vi "InstrumentationU6Mk2.vi"() -> ()   [LabVIEW 2021]
panel:
  out "Waveform Chart 5":dbl(graph)
  out "Waveform Chart 4":dbl(graph)
  out "Waveform Chart 3":dbl(graph)
  out "Waveform Chart 2":dbl(graph)
  out "Waveform Chart":dbl(graph)
  in  "Log Values":bool
  in  "file name":string
  in  "file path":path
  in  "Binary":bool
  in  "SettlingFactor":i32
  in  "Ranges":string[](array[string])=["LJ_rgBIP10V", "LJ_rgBIP10V", "LJ_rgBIPP01V", "LJ_rgBIPP01V"]
  out "Values Read":dbl[](array[numeric]) format="%.6f"
  out "Error Message":string
  in  "Resolution":i32
  out "error out":errorcluster
  # "Aquires multiple analog input channels over USB from the first found U6.\n\nThis uses eAddGoGet from the UD driver, rather than the LabVIEW utility AddS-Go-Get.vi.  The utility\nVI has better/easier error handling and is normally preferred, but eAddGoGet is a single call to the UD driver\nso often preferred if you will have parallel driver calls to the same handle within the same thread (none of\nour examples do this)."
  # "LJ_rgBIP10V\nLJ_rgBIP1V\nLJ_rgBIPP1V\nLJ_rgBIPP01V"
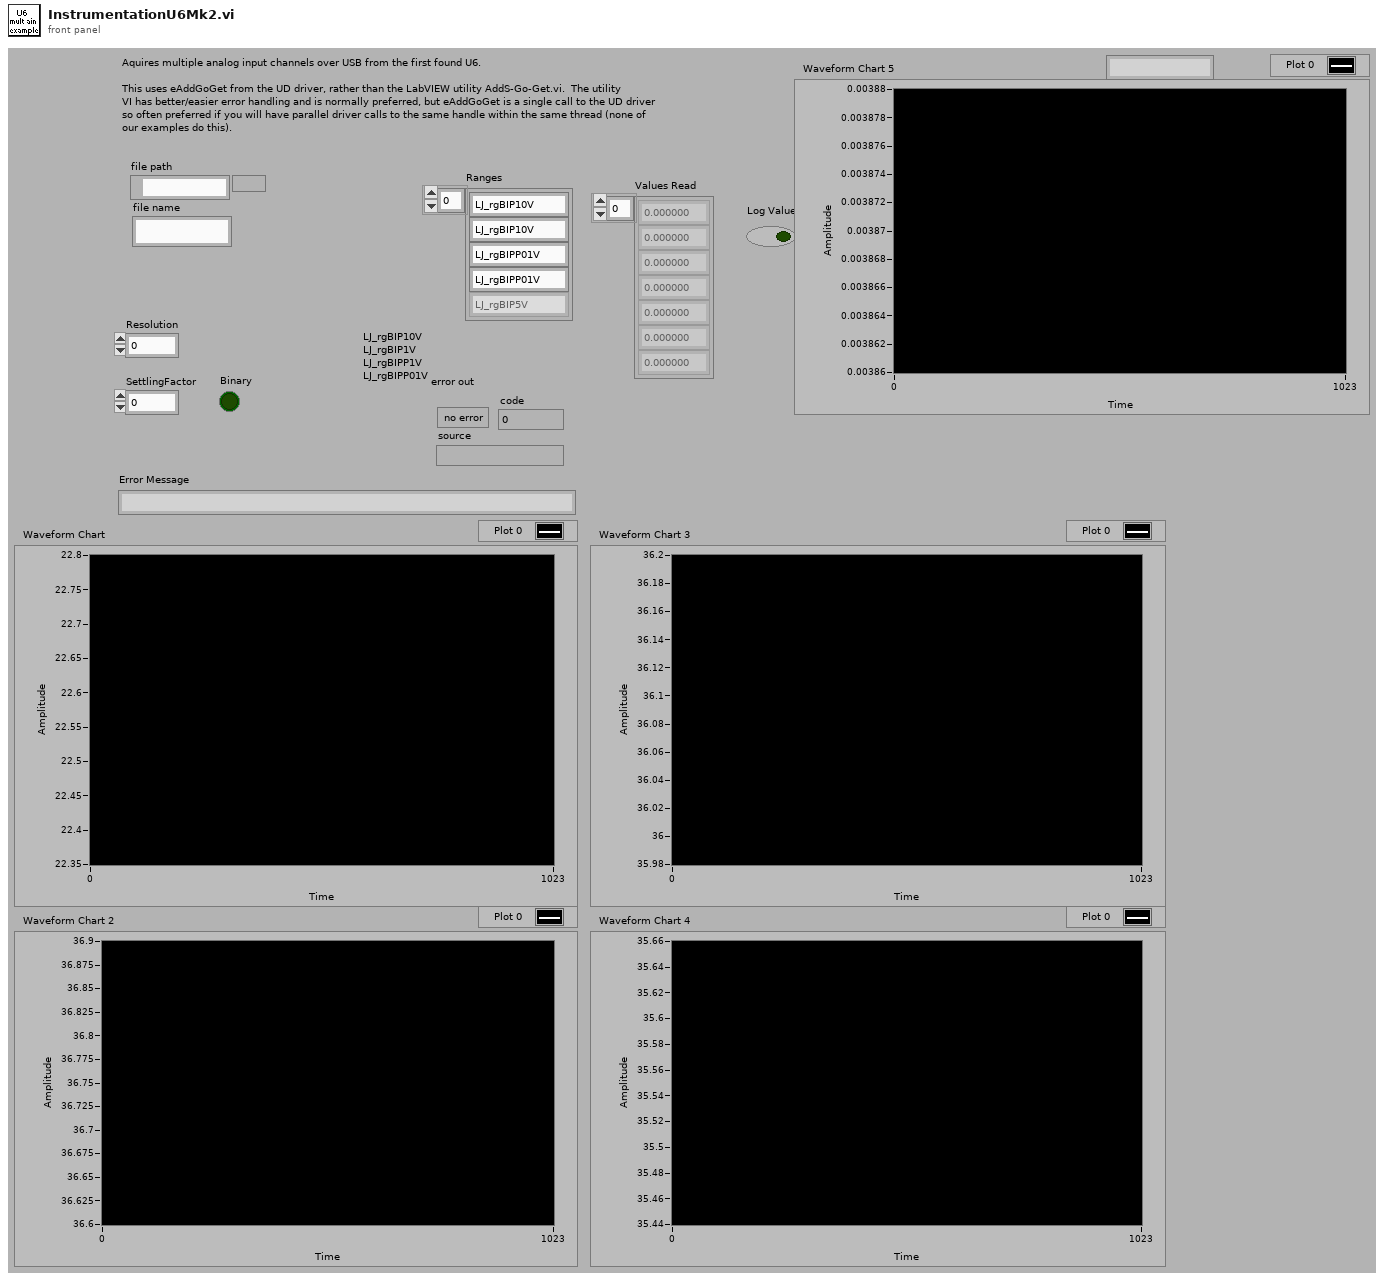
[diagram p1: front panel]
types:
  T1 = enum16{"open", "open or create", "create or replace", "create", "open (read-only)"}
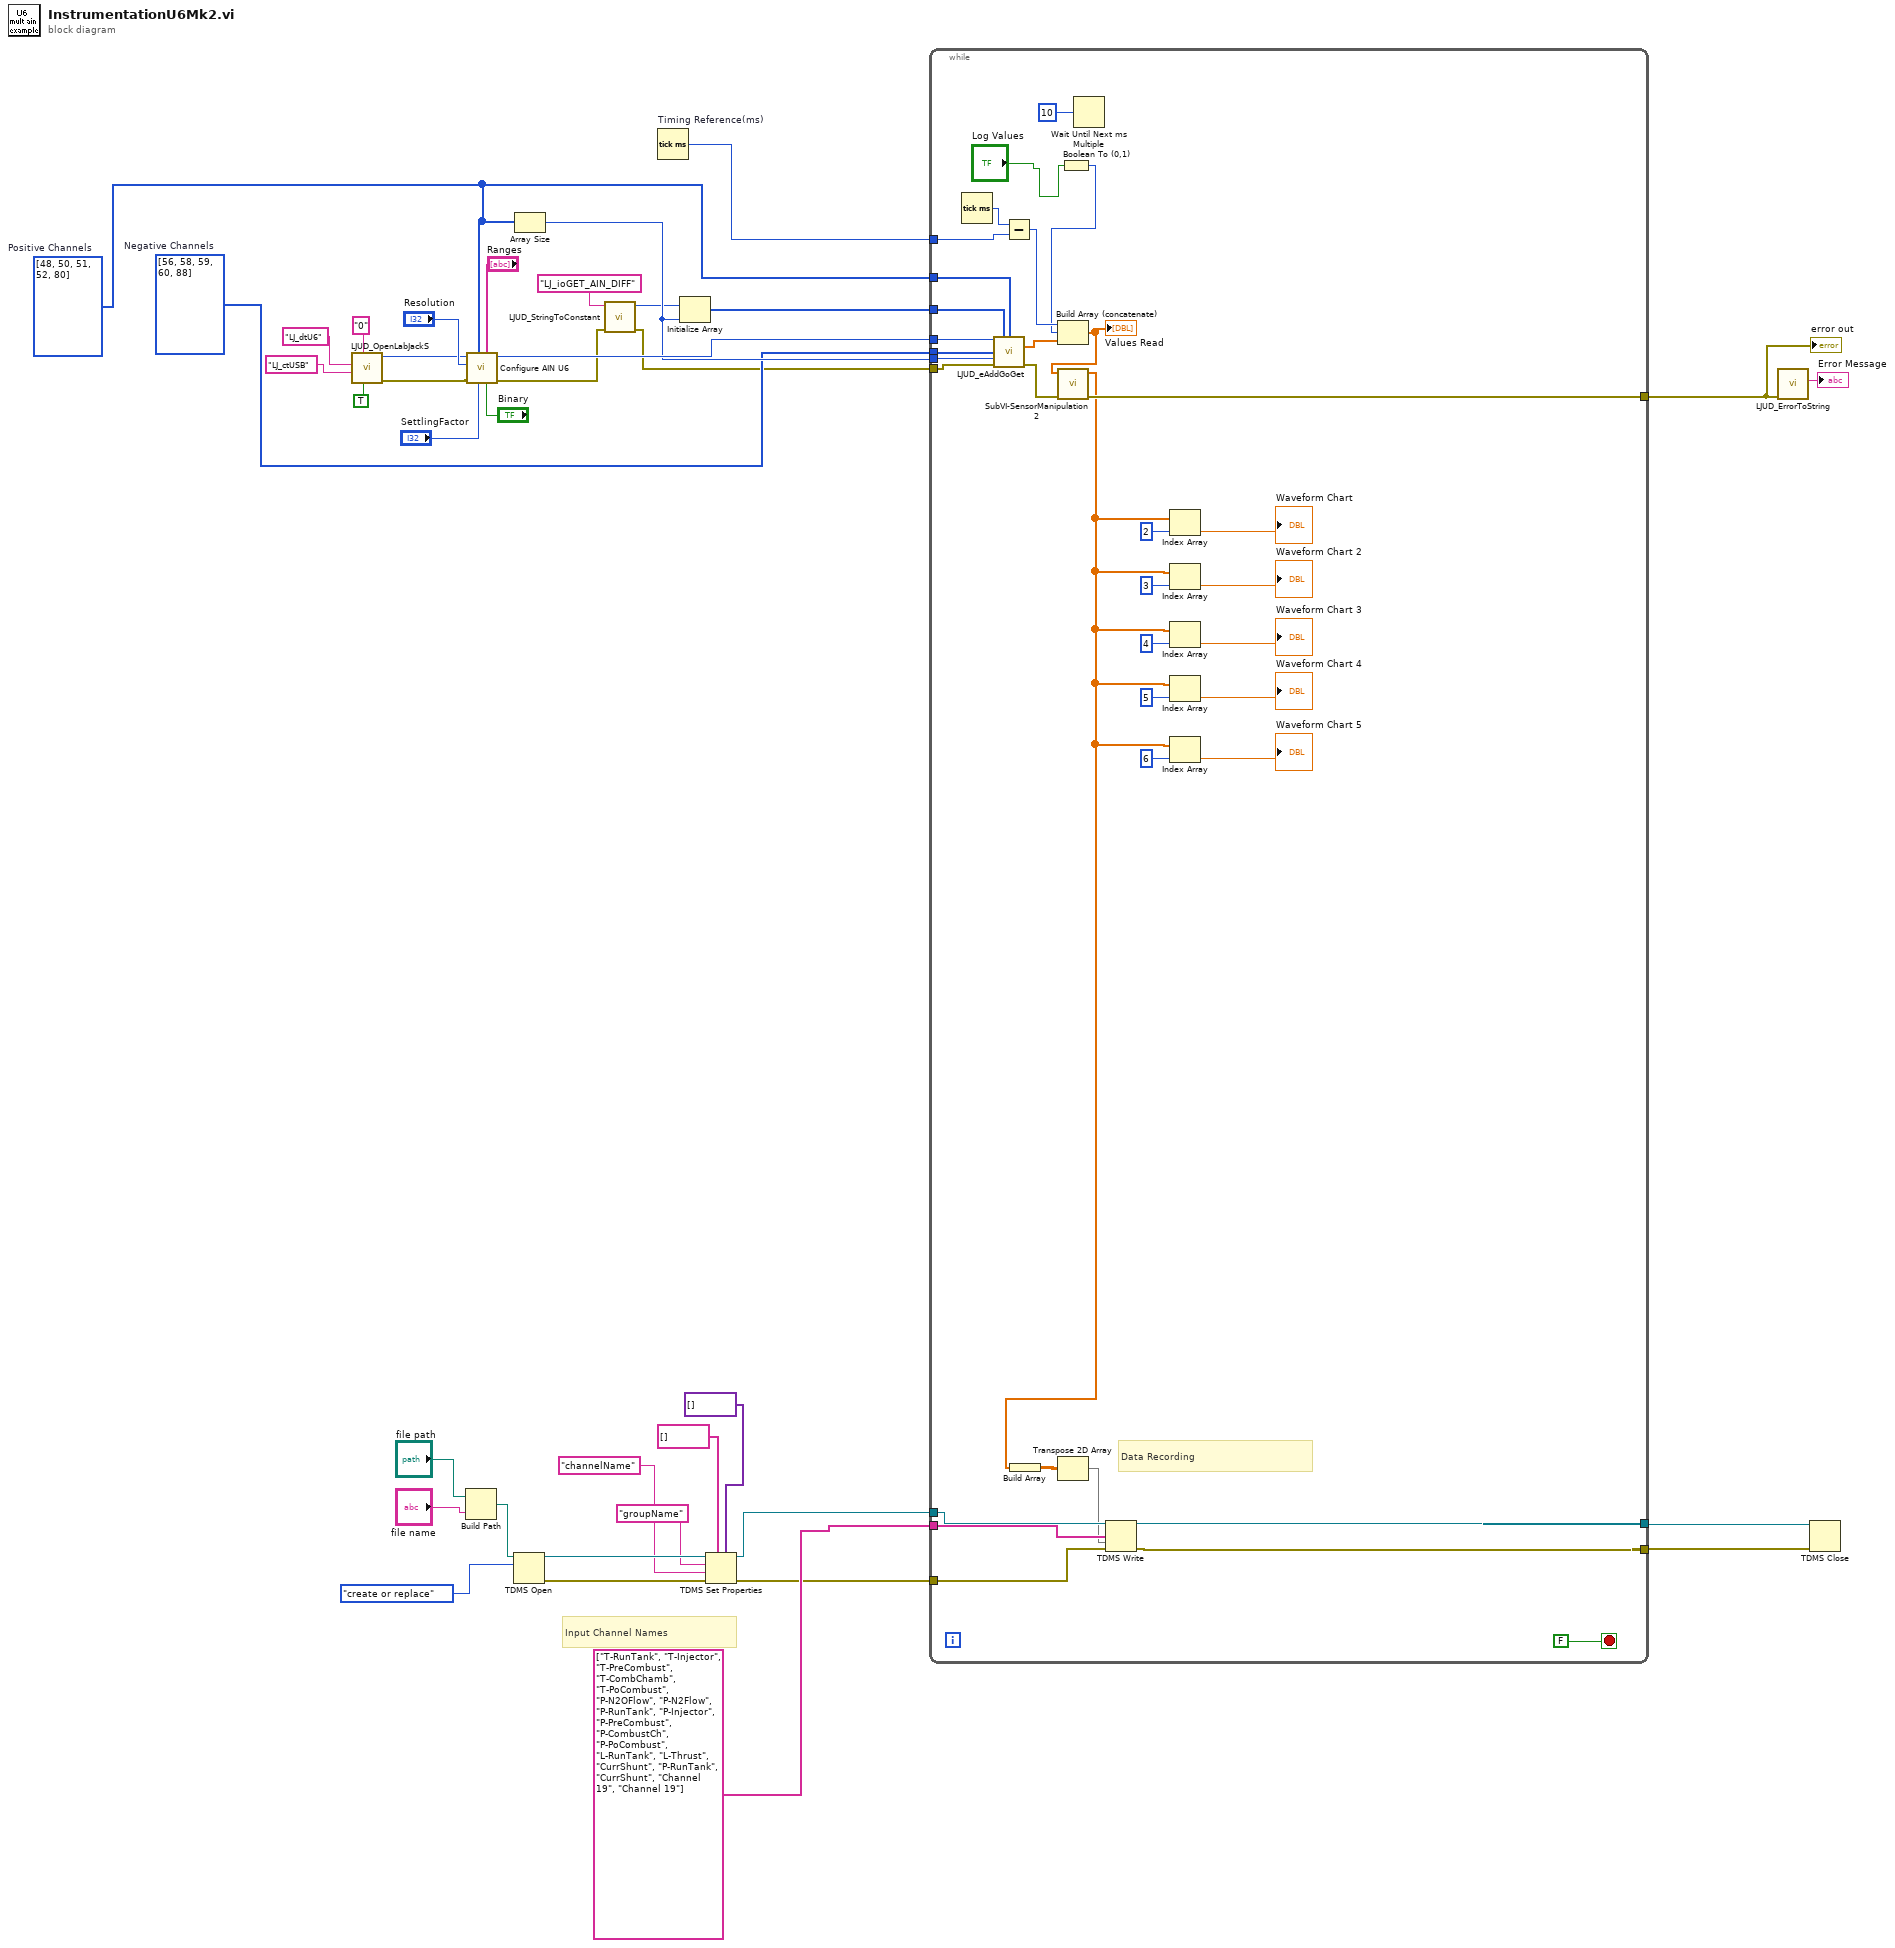
[diagram p0: block diagram]
diagram:
  w19 = i32[] [56, 58, 59, 60, 88]  # Negative Channels
  w18 = i32[] [48, 50, 51, 52, 80]  # Positive Channels
  # "Input Channel Names"
  n1 = call "LJUD_OpenLabJackS.vi"("FirstFound"=TRUE, "Address"="0", "ConnectionType"="LJ_ctUSB", "DeviceType"="LJ_dtU6") -> ("error out"=w28:errorcluster, "Handle"=w29:i32)  [unwired: 5 in, 1 out]
  n2 = Build Path(base path="file path", name or relative path="file name") -> (appended path=w12:path)
  n3 = call "Configure AIN U6.vi"("Binary"="Binary", "Ranges"="Ranges", "SettlingFactor"="SettlingFactor", "Positive Channels"=w18, "error in"=w28, "Resolution"="Resolution", "Handle In"=w29) -> ("error out"=w25:errorcluster, "Handle Out"=w35:i32)  [unwired: 3 in]
  n4 = TDMS Open(10:T1."create or replace" ("operation (0:open)"), 11:w12) -> (0:w17:errorcluster, 3:w16:refnum<k34>)  [unwired: 5 in]
  n5 = Array Size(array=w18) -> (size(s)=w23:i32)
  n6 = call "LJUD_StringToConstant.vi"("error in"=w25, "String"="LJ_ioGET_AIN_DIFF" ("IOType")) -> ("error out"=w1:errorcluster, "Constant Number"=w22:i32)  [unwired: 8 in]
  n7 = Tick Count (ms) "Timing Reference(ms)"() -> (millisecond timer value=w20:u32)
  n8 = Initialize Array(w22, w23) -> (w21:i32[])
  n9 = TDMS Set Properties(5:variant[] [] ("property values"), 7:string[] [] ("property names"), 8:w17, 9:"channelName" ("channel name"), 10:"groupName" ("group name"), 11:w16) -> (0:w5:errorcluster, 3:w7:refnum<k34>)  [unwired: 2 out]
  n10 = while {
    tunnel: w35 -> [w72]
    tunnel: w19 -> [w71]
    tunnel: w23 -> [w70]
    tunnel: w21 -> [w69]
    tunnel: w20 -> [w66]
    tunnel: w18 -> [w64]
    tunnel: w7 -> [w63]
    tunnel: string[] ["T-RunTank", "T-Injector", "T-PreCombust", "T-CombChamb", "T-PoCombust", "P-N2OFlow", "P-N2Flow", "P-RunTank", "P-Injector", "P-PreCombust", "P-CombustCh", "P-PoCombust", "L-RunTank", "L-Thrust", "CurrShunt", "P-RunTank", "CurrShunt", "Channel 19", "Channel 19"] -> [w62]
    tunnel: w5 -> [w61]
    tunnel: [w60] -> w4
    tunnel: [w59] -> w3
    tunnel: [w52] -> w2
    tunnel: w1 -> [w50]
    stop <- FALSE stop-if-true
    # "Data Recording"
    n11 = Tick Count (ms)() -> (millisecond timer value=w67:u32)
    n12 = call "LJUD_eAddGoGet.vi"("Handle In"=w72, "aIOTypes"=w69, "aChannels"=w64, "ax1s"=w71, "NumRequests"=w70, "error in"=w50) -> ("Values Read"=w55:dbl[], "error out"=w51:errorcluster)  [unwired: 4 in, 4 out]
    n13 = Subtract(x=w67, y=w66) -> (x-y=w65:u32)
    n14 = Boolean To (0,1)(Boolean="Log Values") -> (0, 1=w54:i16)
    n15 = Build Array (concatenate)(w65, w54, w55) -> (w53:dbl[])
    "Values Read" <- w53
    n16 = call "SubVI-SensorManipulation2.vi"("error in"=w51, "Array in"=w53) -> ("error out"=w52:errorcluster, "Array out"=w39:dbl[])  [unwired: 8 in]
    n17 = Build Array(w39) -> (w57:dbl[][])
    n18 = Transpose 2D Array(2D array=w57) -> (transposed array=w56:dbl[][])
    n19 = Wait Until Next ms Multiple(millisecond multiple=u32 10) -> ()  [unwired: 1 out]
    n20 = TDMS Write(0:w63, 7:w62, 9:w56, 11:w61) -> (4:w59:refnum<k34>, 15:w60:errorcluster)  [unwired: 2 in, 2 out]
    n21 = Index Array(array=w39, index=2) -> (element=→"Waveform Chart":dbl)
    n22 = Index Array(array=w39, index=3) -> (element=→"Waveform Chart 2":dbl)
    n23 = Index Array(array=w39, index=4) -> (element=→"Waveform Chart 3":dbl)
    n24 = Index Array(array=w39, index=5) -> (element=→"Waveform Chart 4":dbl)
    n25 = Index Array(array=w39, index=6) -> (element=→"Waveform Chart 5":dbl)
  }
  "error out" <- w2
  n26 = call "LJUD_ErrorToString.vi"("error in"=w2) -> ("String"=→"Error Message":string)  [unwired: 10 in]
  n27 = TDMS Close(8:w4, 11:w3) -> ()  [unwired: 2 out]
